vi "comm.vi"(8 "error in (no error)":errorcluster, 11 "UI Actor in":refnum<class "UI Actor.lvclass">) -> (0 "error out":errorcluster, 2 "Comando Out":string, 3 "UI Actor out":refnum<class "UI Actor.lvclass">)   [LabVIEW 2020]
uses:
  UI Actor.lvclass
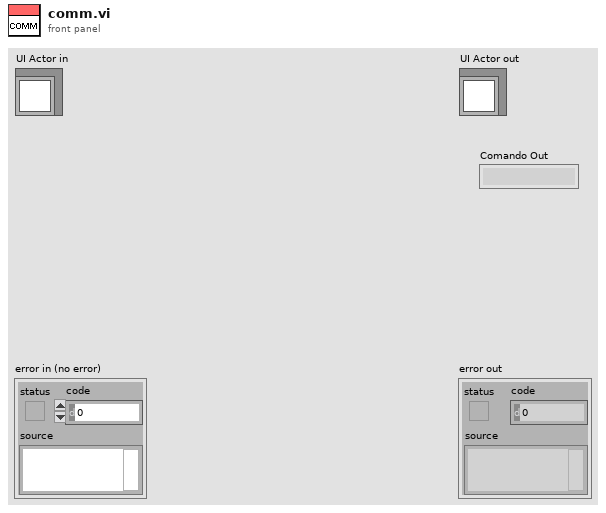
[diagram p1: front panel]
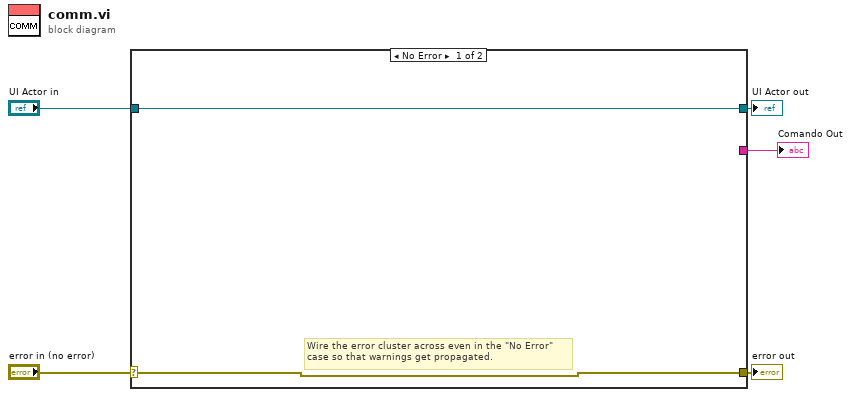
[diagram p0: block diagram]
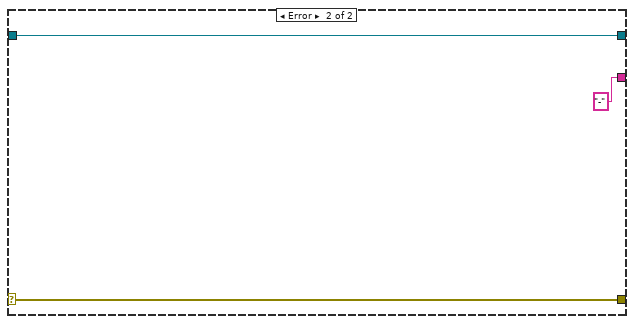
[diagram p2: hidden frame]
diagram:
  n1 = case shown="No Error" "error in (no error)" {
    selector: "error in (no error)" -> [w6 w10]
    tunnel: [w6 w10] -> w4
    tunnel: [w7 w9] -> w2
    tunnel: "UI Actor in" -> [w7 w9]
    tunnel: [_ "-" ("Comando")] -> w1
    frame No Error {
      # "Wire the error cluster across even in the \"No Error\"\ncase so that warnings get propagated."
    }
    frame Error {
    }
  }
  "error out" <- w4
  "UI Actor out" <- w2
  "Comando Out" <- w1
